vi "Graph_Output_v00.vi"(8 "Outputs":T2, 11 "Safety First":T1) -> ()   [LabVIEW 2010]
doc: "Outputs the signals to FPGA output nodes, after a variable rate-limiter has been applied."
uses:
  Strict Type Defs/Graph Output.ctl
  Strict Type Defs/Safety First.ctl
  <vilib>/rvi/Analysis/common/polyVINode/niFpgaPolyViWrapper.xnode
  <vilib>/eio/EIONode/EIONode.xnode
  <vilib>/rvi/eio/nirviEIOImplementation/nirviEIOImplementation.xnode
  <vilib>/rvi/eio/common/nirviEmuClasses.ctl
  <vilib>/express/rvi/analysis/control/nonlinear/niFPGA Rate Limiter.vi
  <vilib>/express/rvi/analysis/control/nonlinear/niFPGA Rate Limiter (I16).vi
  <vilib>/rvi/eio/common/nirviEmuTemplateMethod_noerrors.vi
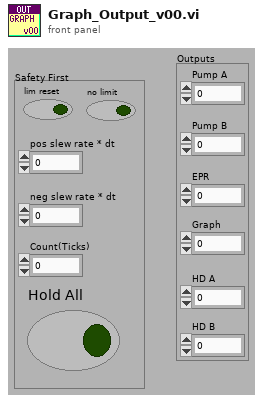
[diagram p1: front panel]
types:
  T1 = typedef "Safety First.ctl" = cluster{"lim reset":bool, "no limit":bool, "pos slew rate * dt":i16, "neg slew rate * dt":i16, "Hold All":bool, "Count(Ticks)":u32}
  T2 = typedef "Graph Output.ctl" = cluster{"Pump A":i16, "Pump B":i16, "EPR":i16, "Graph":i16, "HD A":i16, "HD B":i16}
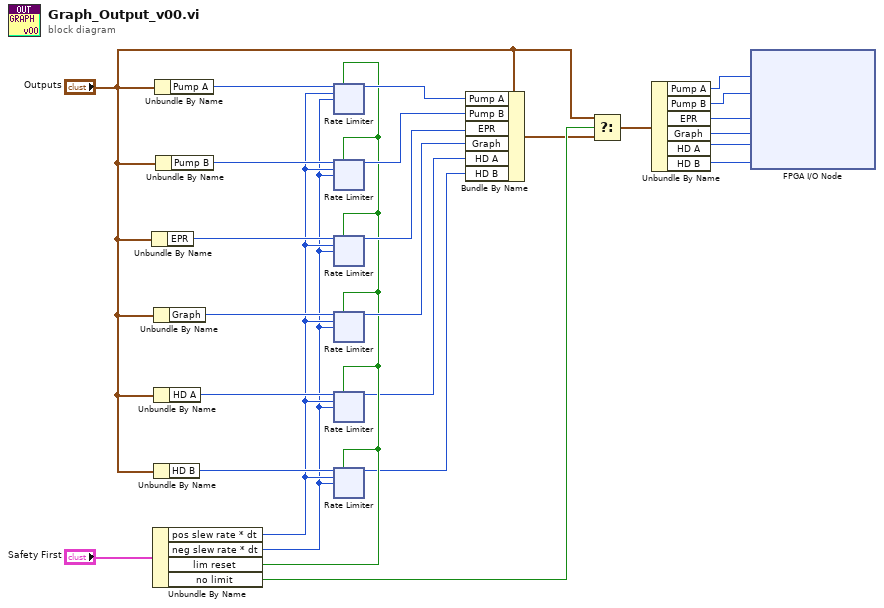
[diagram p0: block diagram]
diagram:
  n1 = Unbundle By Name("Outputs") -> ("EPR"=w23:i16)
  n2 = Unbundle By Name("Safety First") -> ("pos slew rate * dt"=w4:i16, "neg slew rate * dt"=w3:i16, "lim reset"=w5:bool, "no limit"=w17:bool)
  n3 = Unbundle By Name("Outputs") -> ("Graph"=w22:i16)
  n4 = Unbundle By Name("Outputs") -> ("HD A"=w7:i16)
  n5 = Unbundle By Name("Outputs") -> ("HD B"=w8:i16)
  n6 = Unbundle By Name("Outputs") -> ("Pump A"=w25:i16)
  n7 = Unbundle By Name("Outputs") -> ("Pump B"=w24:i16)
  n8 = xnode "Rate Limiter"("pos slew rate * dt"=w4, "input"=w25, "neg slew rate * dt"=w3, "reset"=w5) -> ("output"=w21:i16)
  n9 = xnode "Rate Limiter"("pos slew rate * dt"=w4, "input"=w24, "neg slew rate * dt"=w3, "reset"=w5) -> ("output"=w20:i16)
  n10 = xnode "Rate Limiter"("pos slew rate * dt"=w4, "input"=w23, "neg slew rate * dt"=w3, "reset"=w5) -> ("output"=w19:i16)
  n11 = xnode "Rate Limiter"("pos slew rate * dt"=w4, "input"=w22, "neg slew rate * dt"=w3, "reset"=w5) -> ("output"=w18:i16)
  n12 = xnode "Rate Limiter"("pos slew rate * dt"=w4, "input"=w7, "neg slew rate * dt"=w3, "reset"=w5) -> ("output"=w2:i16)
  n13 = xnode "Rate Limiter"("pos slew rate * dt"=w4, "input"=w8, "neg slew rate * dt"=w3, "reset"=w5) -> ("output"=w1:i16)
  n14 = Bundle By Name(cluster="Outputs", "Pump A"=w21, "Pump B"=w20, "EPR"=w19, "Graph"=w18, "HD A"=w2, "HD B"=w1) -> (w11:T2)
  n15 = Select(t="Outputs", s=w17, f=w11) -> (s? t:f=w16:T2)
  n16 = Unbundle By Name(w16) -> ("Pump A"=w15:i16, "Pump B"=w14:i16, "EPR"=w13:i16, "Graph"=w12:i16, "HD A"=w10:i16, "HD B"=w9:i16)
  n17 = xnode "FPGA I/O Node"("Connector0/AO0"=w15, "Connector0/AO1"=w14, "Connector0/AO2"=w13, "Connector0/AO3"=w12, "Connector0/AO4"=w10, "Connector0/AO5"=w9) -> ()  [unwired: 6 in, 6 out]
